vi "Process.vi"(8 "error in":errorcluster, 11 "Render.IMAQ":refnum<class "Render.IMAQ.lvclass">) -> (0 "error out":errorcluster, 3 "Render.IMAQ out":refnum<class "Render.IMAQ.lvclass">)   [LabVIEW 2019, in "Render.IMAQ.lvclass"]
doc: "---------------------------------------------------------------\nJKI State Machine Objects™\nhttp://jki.net/state-machine-objects/\nCopyright (C) 2005-2015, JKI <info@jki.net>\nALL RIGHTS RESERVED"
uses:
  Render.IMAQ.lvclass
  C:/Program Files (x86)/National Instruments/LabVIEW 2019/vi.lib/JKI/JKI SMO/SMO/SMO.lvclass
  <userlib>/LevyLab/Relay Box/Typedefs/Resistor--enum.ctl
  <vilib>/JKI/JKI SMO/SMO/Typedefs/Parent Call--Enum.ctl
  <vilib>/vision/Image Controls.llb/IMAQ Image.ctl
  <vilib>/JKI/JKI SMO/SMO/SMO.lvclass/SMO.ctl
  Render.IMAQ.lvclass/Render.IMAQ.ctl
  <vilib>/JKI/JKI SMO/SMO/Private/ReftoDVR--SMO.vi
  <vilib>/JKI/JKI SMO/SMO/SMO.lvclass
  <userlib>/LevyLab/Relay Box/Relay-Box.lvclass
panel:
  out "Array 2":T2(array[cluster])
  out "New Litho Data":T2(array[cluster])
  out "Array":bool[](array[boolean])
  # "For instructions on how to use the JKI State Machine Objects, examples and video tutorials, visit:\nhttp://jki.net/state-machine-objects/\n\nJKI State Machine Objects™\nhttp://jki.net/state-machine-objects/\nCopyright (C) 2005-2015, JKI <info@jki.net>\nALL RIGHTS RESERVED"
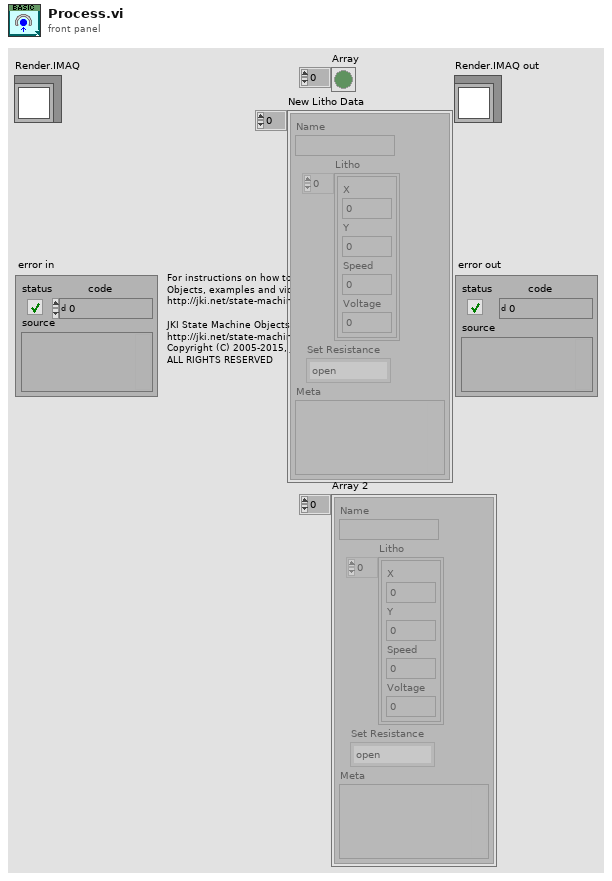
[diagram p1: front panel]
types:
  T1 = typedef "Relay-Box.lvclass/Resistor--enum.ctl" = enum16{"open", "discharge tip", "0 ohms", "100k ohm", "10M ohm", "1G ohm"}
  T2 = cluster{"Name":string, "Litho":cluster{"X":dbl, "Y":dbl, "Speed":dbl, "Voltage":dbl}[], "Set Resistance":T1, "Meta":variant}[]
  T3 = typedef "SMO.lvclass/Parent Call--Enum.ctl" = enum16{"Allows parent to run", "Does not request parent to run"}
  T4 = enum32{"invalid app kind", "Development System", "Run Time System", "Student Edition", "Embedded LabVIEW", "Evaluation", "Custom"}
  T5 = enum32{"Invalid", "Standard", "Closed", "Hidden", "Minimized", "Maximized"}
  T6 = enum32{"Bad", "Idle", "Run top level", "Running"}
  T7 = typedef "Render.IMAQ.lvclass/PrivateEvents--Render.IMAQ.New Background Image.ctl" = path
  T8 = typedef "IMAQ Image.ctl" = refnum<image>
  T9 = cluster{"Core":cluster{"Current VI Reference":refnum<vi>, "Close Panel on Exit?":bool, "error":errorcluster}, "Self Reference":refnum<class "Render.IMAQ.lvclass">, "Your string data":string, "Litho Data":cluster{"Name":string, "Litho":cluster{"X":dbl, "Y":dbl, "Speed":dbl, "Voltage":dbl}[], "Set Resistance":T1, "Meta":variant}[], "New Litho Data":cluster{"Name":string, "Litho":cluster{"X":dbl, "Y":dbl, "Speed":dbl, "Voltage":dbl}[], "Set Resistance":T1, "Meta":variant}[], "Background Path":path, "Changed":cluster{"Found":bool[], "Data":cluster{"Name":string, "Litho":cluster{"X":dbl, "Y":dbl, "Speed":dbl, "Voltage":dbl}[], "Set Resistance":T1, "Meta":variant}[]}, "IMAQ Work":T8}
  T10 = typedef "Render.IMAQ.lvclass/PrivateEvents--Render.IMAQ.NewLithographyData.ctl" = variant
  T11 = cluster{"Found":bool[], "Data":cluster{"Name":string, "Litho":cluster{"X":dbl, "Y":dbl, "Speed":dbl, "Voltage":dbl}[], "Set Resistance":T1, "Meta":variant}[]}
  T12 = cluster{"Current VI Reference":refnum<vi>, "Close Panel on Exit?":bool, "error":errorcluster}
  T13 = typedef "SMO.lvclass/Protected Events.ctl" = cluster{"StopProcesses":refnum<user-event>, "AbortProcesses":refnum<user-event>, "Config Changed":refnum<user-event>, "Dependency":refnum<user-event>}
  T14 = typedef "Render.IMAQ.lvclass/PrivateEvents--Cluster.ctl" = cluster{"New Background Image":refnum<user-event>, "NewLithographyData":refnum<user-event>}
  T15 = cluster{"Name":string, "Litho":cluster{"X":dbl, "Y":dbl, "Speed":dbl, "Voltage":dbl}[], "Set Resistance":T1, "Meta":variant}
  T16 = typedef "Image Type" = u32
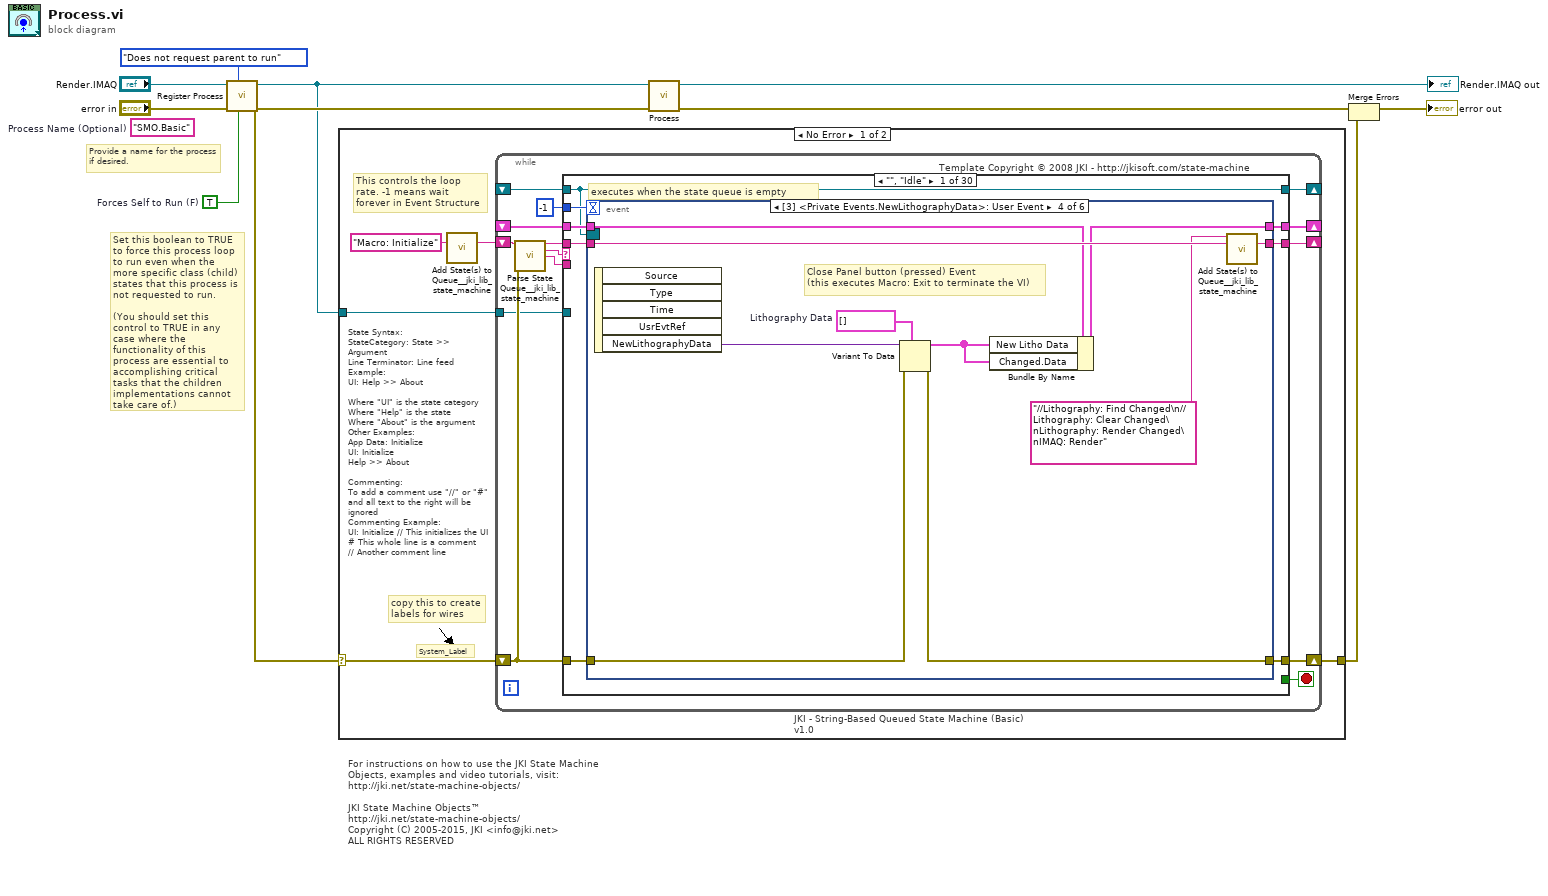
[diagram p0: block diagram]
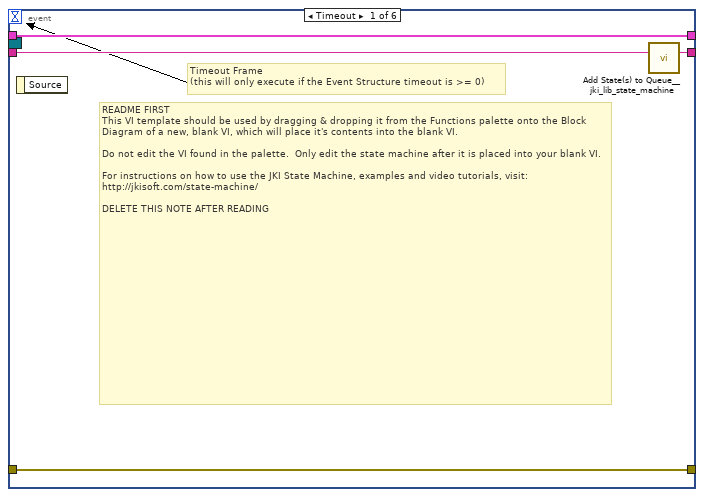
[diagram p2: hidden frame]
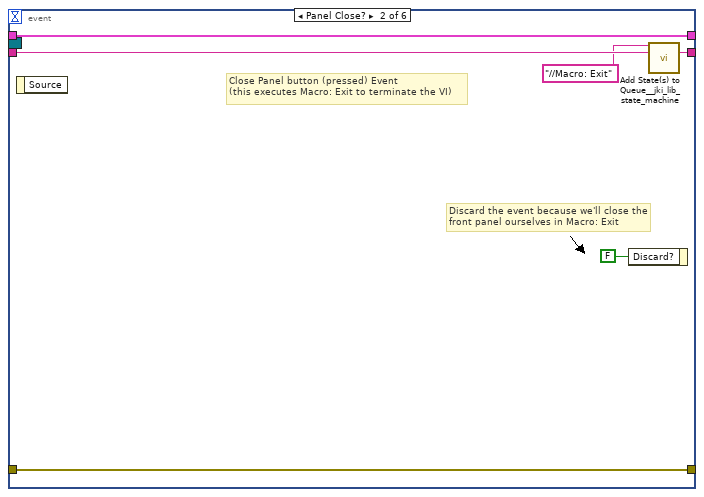
[diagram p3: hidden frame]
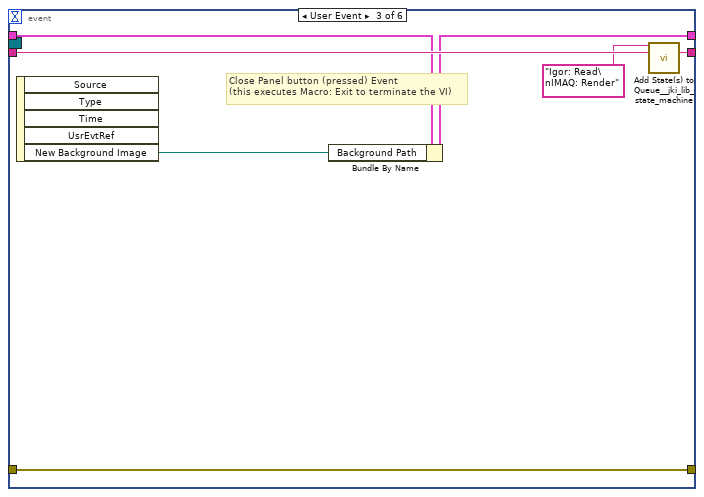
[diagram p4: hidden frame]
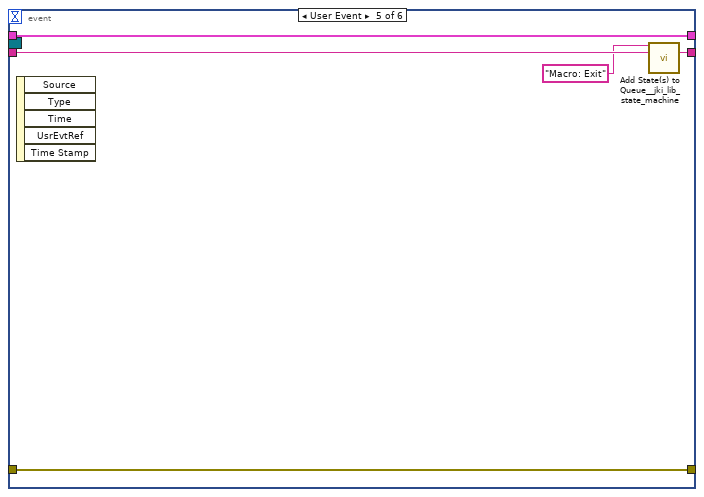
[diagram p5: hidden frame]
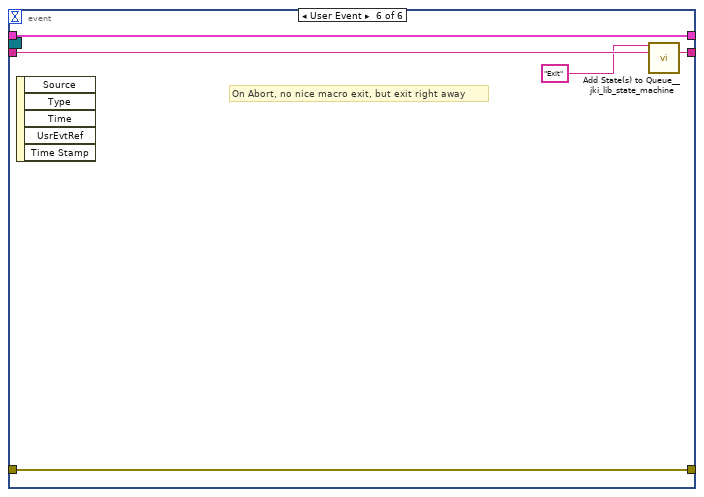
[diagram p6: hidden frame]
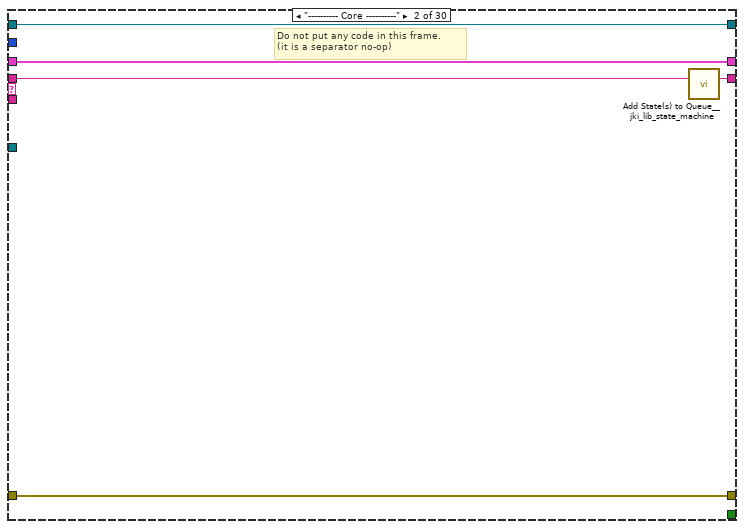
[diagram p7: hidden frame]
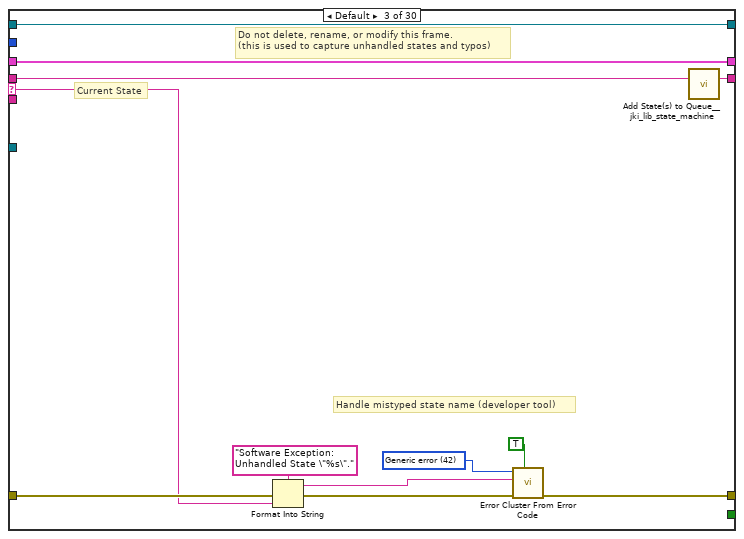
[diagram p8: hidden frame]
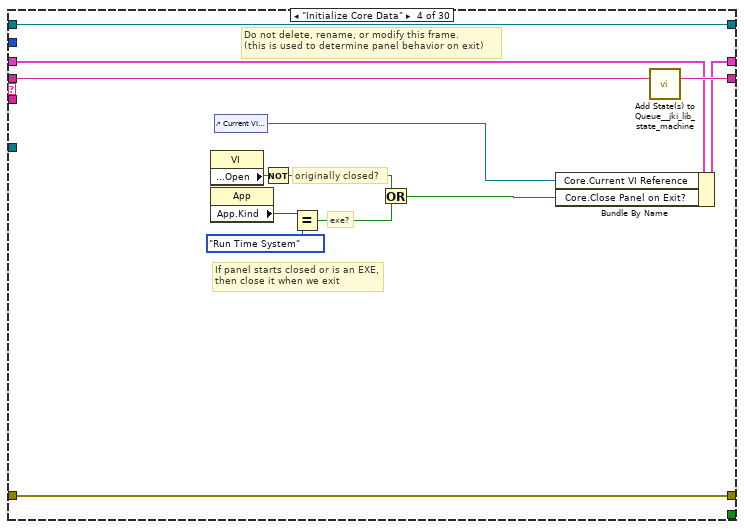
[diagram p9: hidden frame]
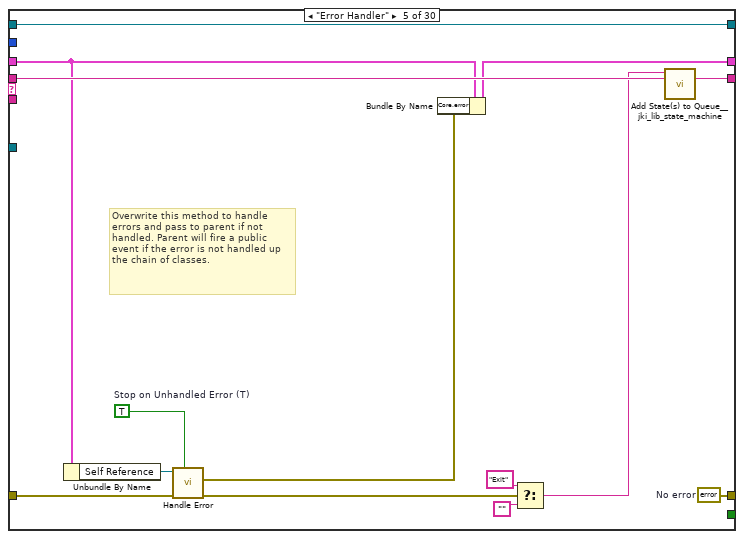
[diagram p10: hidden frame]
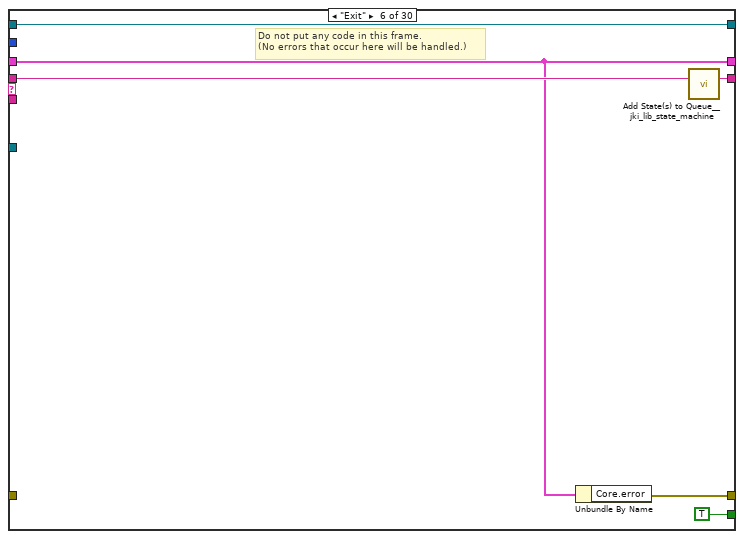
[diagram p11: hidden frame]
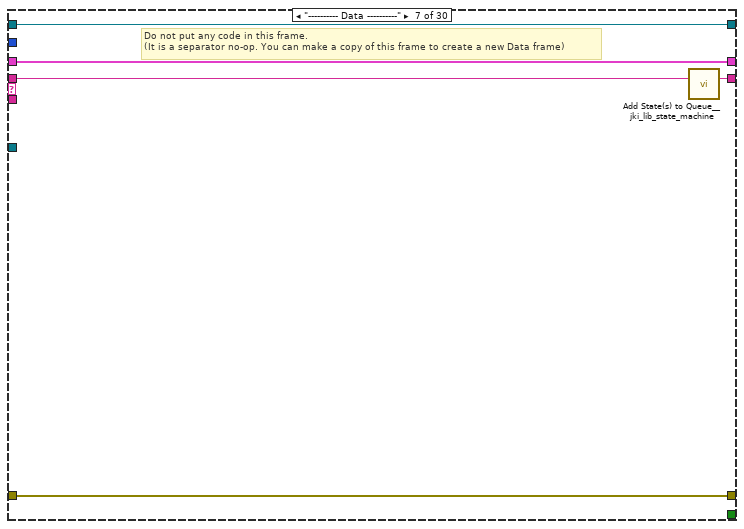
[diagram p12: hidden frame]
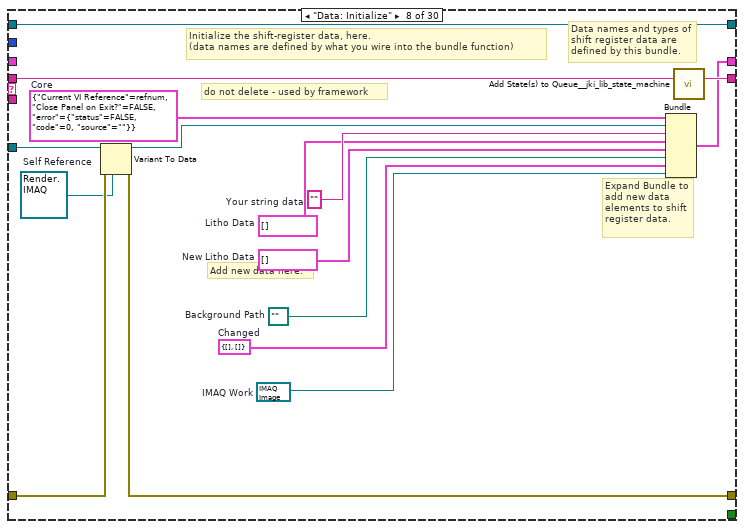
[diagram p13: hidden frame]
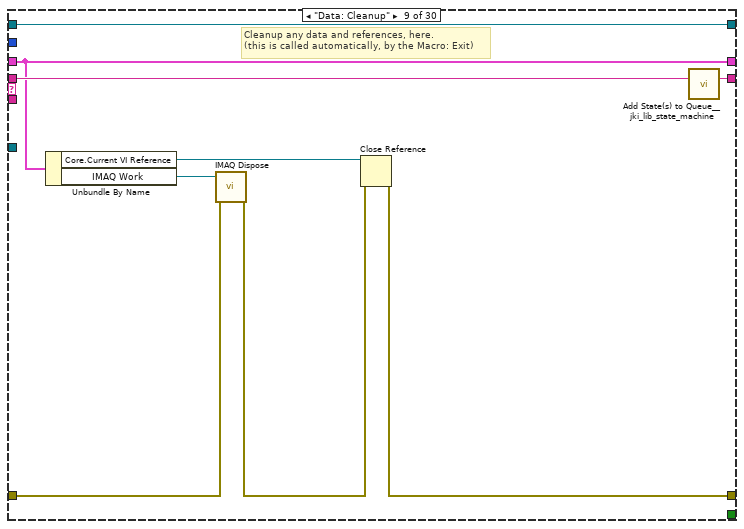
[diagram p14: hidden frame]
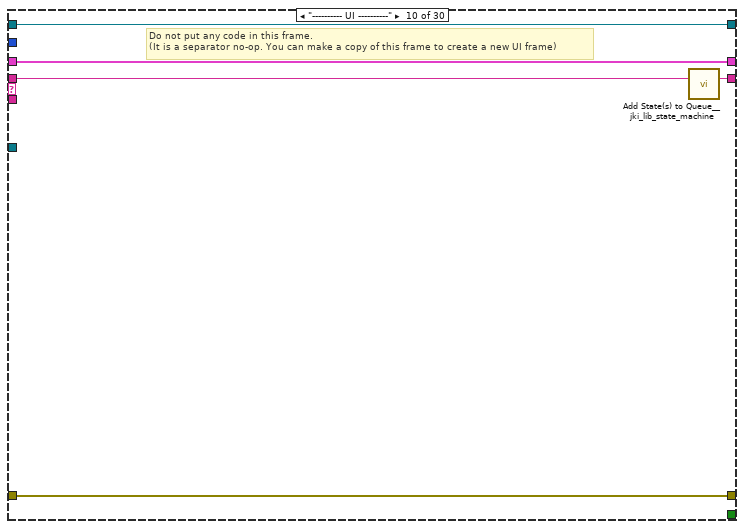
[diagram p15: hidden frame]
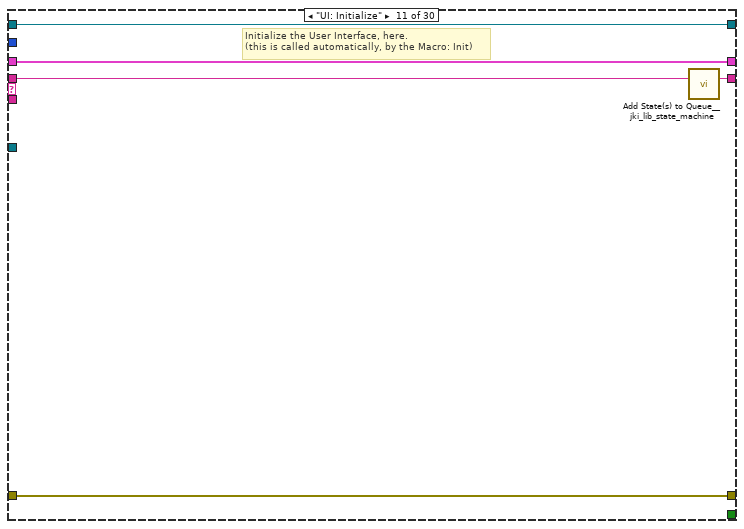
[diagram p16: hidden frame]
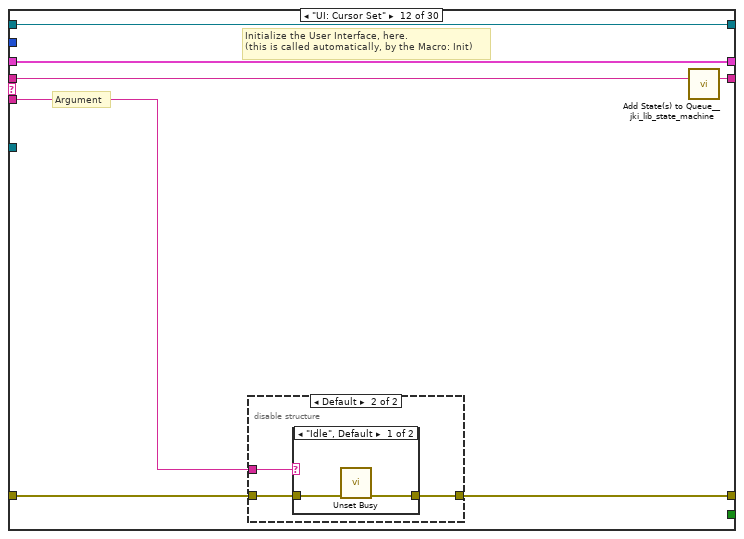
[diagram p17: hidden frame]
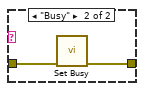
[diagram p19: hidden frame]
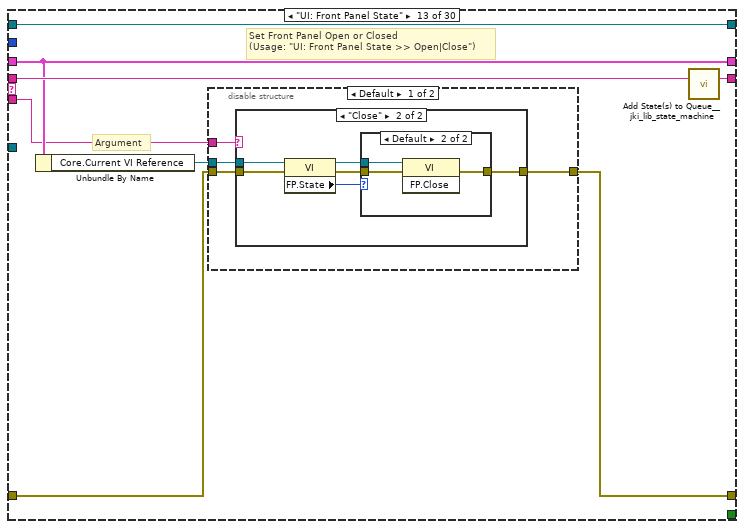
[diagram p20: hidden frame]
diagram:
  w1 = TRUE  # Forces Self to Run (F)
  (unwired) "SMO.Basic"  # Process Name (Optional)
  # "Provide a name for the process\nif desired."
  # "Set this boolean to TRUE to force this process loop to run even when the more specific class (child) states that this process is not requested to run.\n\n(You should set this control to TRUE in any case where the functionality of this process are essential to accomplishing critical tasks that the children implementations cannot take care of.)"
  # "For instructions on how to use the JKI State Machine Objects, examples and video tutorials, visit:\nhttp://jki.net/state-machine-objects/\n\nJKI State Machine Objects™\nhttp://jki.net/state-machine-objects/\nCopyright (C) 2005-2015, JKI <info@jki.net>\nALL RIGHTS RESERVED"
  n1 = call <vilib>:"Register Process.vi"("Forces Self to Run (F)"=w1, "Parent Call"=Parent_Call--Enum."Does not request parent to run", "error in (no error)"="error in", "SMO"="Render.IMAQ") -> ("error out"=w7:errorcluster, "SMO out"=w6:refnum<class "Render.IMAQ.lvclass">)  [unwired: 6 in]
  n2 = case shown="No Error" w7 {
    selector: w7 -> [w12 w397]
    tunnel: w6 -> [w13 _]
    tunnel: [w11 w397] -> w3
    frame No Error {
      # "State Syntax:\nStateCategory: State >> Argument\nLine Terminator: Line feed\nExample:\nUI: Help >> About\n\nWhere \"UI\" is the state category\nWhere \"Help\" is the state\nWhere \"About\" is the argument\nOther Examples:\nApp Data: Initialize\nUI: Initialize\nHelp >> About\n\nCommenting:\nTo add a comment use \"//\" or \"#\" and all text to the right will be ignored\nCommenting Example:\nUI: Initialize // This initializes the UI\n# This whole line is a comment\n// Another comment line"
      # "copy this to create labels for wires"
      # "This controls the loop rate. -1 means wait forever in Event Structure"
      # "System_Label"
      n3 = call <vilib>:"Add State(s) to Queue__jki_lib_state_machine.vi"("State(s) in (\"\")"="Macro: Initialize") -> ("States Out"=w15:string)  [unwired: 14 in]
      n4 = while "JKI - String-Based Queued State Machine (Basic) v1.0" {
        shift-right: [w22] -> _
        shift-left: _ -> [w21]
        shift-right: [w25] -> w11
        shift-left: w12 -> [w19]
        shift-right: [w24] -> _
        shift-left: w15 -> [w26]
        tunnel: w13 -> [w18]
        shift-right: [w17] -> _
        shift-left: _ -> [w16]
        stop <- w23 stop-if-true
        # "Template Copyright © 2008 JKI - http://jkisoft.com/state-machine"
        n5 = call <vilib>:"Parse State Queue__jki_lib_state_machine.vi"("State Queue"=w26, "Error In (no error)"=w19) -> ("Remaining States"=w28:string, "Current State"=w29:string, "Arguments"=w27:string)  [unwired: 11 in]
        n6 = case shown="\"\", \"Idle\"" w29 {
          selector: w29 -> [_ _ w81 _ _ _ _ _ _ _ _ _ _ _ _ _ _ _ _ _ _ _ _ _ _ _ _ _ _ _]
          tunnel: w28 -> [w37 w79 w85 w104 w118 w124 w129 w145 w154 w159 w164 w171 w187 w219 w233 w247 w252 w263 w268 w280 w286 w291 w303 w314 w344 w359 w369 w378 w383 w396]
          tunnel: w27 -> [_ _ _ _ _ _ _ _ _ _ _ w165 w181 _ _ _ _ _ _ _ _ _ _ _ _ _ _ _ _ _]
          tunnel: w21 -> [w35 w76 w83 w95 w112 w120 w126 _ w150 w156 w162 w169 w183 w216 w229 w238 w249 w260 w265 w278 w284 w289 w295 w309 w336 w357 w360 w375 w381 w386]
          tunnel: [w34 w77 w87 w101 w113 w119 w127 w140 w151 w157 w161 w166 w184 w217 w231 w245 w250 w254 w266 w274 w282 w287 w294 w311 w339 w355 w365 w370 w379 w392] -> w25
          tunnel: w19 -> [w33 w77 w86 w101 w114 _ w127 w141 w146 w157 w161 w167 w185 w217 w231 w245 w250 w255 w266 w275 w282 w287 w293 w311 w338 w355 w364 w371 w379 w391]
          tunnel: [w36 w78 w84 w103 w117 w123 w128 w144 w153 w158 w163 w170 w186 w218 w232 w246 w251 w262 w267 w279 w285 w290 w302 w313 w343 w358 w368 w377 w382 w395] -> w24
          tunnel: [_ _ _ _ _ TRUE _ _ _ _ _ _ _ _ _ _ _ _ _ _ _ _ _ _ _ _ _ _ _ _] -> w23
          tunnel: [w32 w76 w83 w102 w111 w120 w126 w143 w150 w156 w162 w169 w183 w216 w229 w238 w249 w260 w265 w278 w284 w289 w296 w310 w337 w357 w361 w375 w381 w387] -> w22
          tunnel: -1 ("Timeout") -> [w31 _ _ _ _ _ _ _ _ _ _ _ _ _ _ _ _ _ _ _ _ _ _ _ _ _ _ _ _ _]
          tunnel: w18 -> [_ _ _ _ _ _ _ w138 _ _ _ _ _ _ _ _ _ _ _ _ _ _ _ _ _ _ _ _ _ _]
          tunnel: [w30 w75 w80 w92 w116 w121 w125 w136 w149 w155 w160 w168 w180 w215 w230 w239 w248 w261 w264 w277 w283 w288 w301 w312 w342 w356 w367 w376 w380 w394] -> w17
          tunnel: w16 -> [w30 w75 w80 w92 w116 w121 w125 w136 w149 w155 w160 w168 w180 w215 w230 w239 w248 w261 w264 _ w283 w288 w301 w312 w342 w356 w367 w376 w380 w394]
          frame "", "Idle" {
            # "executes when the state queue is empty"
            n7 = event shown="[3] <Private Events.NewLithographyData>: User Event" {
              selector: w30 -> [_ _ _ _ _ _]
              dyn-events: _ -> [_ _ _ _ _ _]
              timeout: w31 -> [_ _ _ _ _ _]
              tunnel: w37 -> [w41 w47 w54 w64 w69 w74]
              tunnel: [w40 w46 w53 w63 w68 w73] -> w36
              tunnel: w35 -> [w39 w44 w49 w56 w66 w71]
              tunnel: [w38 w45 w52 w60 w67 w72] -> w34
              tunnel: w33 -> [w38 w45 w52 w59 w67 w72]
              tunnel: [w39 w44 w50 w57 w66 w71] -> w32
              event Timeout {
                # "README FIRST\nThis VI template should be used by dragging & dropping it from the Functions palette onto the Block Diagram of a new, blank VI, which will place it's contents into the blank VI.\n\nDo not edit the VI found in the palette.  Only edit the state machine after it is placed into your blank VI.\n\nFor instructions on how to use the JKI State Machine, examples and video tutorials, visit:\nhttp://jkisoft.com/state-machine/\n\nDELETE THIS NOTE AFTER READING"
                # "Timeout Frame\n(this will only execute if the Event Structure timeout is >= 0)"
                n8 = event-data() -> ()  [unwired: 1 in, 1 out]
                n9 = call <vilib>:"Add State(s) to Queue__jki_lib_state_machine.vi"("State(s) in (\"\")"=w41) -> ("States Out"=w40:string)  [unwired: 14 in]
              }
              event Panel Close? {
                # "Discard the event because we'll close the front panel ourselves in Macro: Exit"
                # "Close Panel button (pressed) Event\n(this executes Macro: Exit to terminate the VI)"
                n10 = event-data() -> ()  [unwired: 1 in, 1 out]
                n11 = event-data("Discard?"=FALSE) -> ()  [unwired: 1 in, 1 out]
                n12 = call <vilib>:"Add State(s) to Queue__jki_lib_state_machine.vi"("State(s) in Front (\"\")"="//Macro: Exit", "State(s) in (\"\")"=w47) -> ("States Out"=w46:string)  [unwired: 13 in]
              }
              event User Event {
                # "Close Panel button (pressed) Event\n(this executes Macro: Exit to terminate the VI)"
                n13 = event-data() -> ("New Background Image"=w48:T7)  [unwired: 1 in, 4 out]
                n14 = Bundle By Name(cluster=w49, "Background Path"=w48) -> (w50:T9)
                n15 = call <vilib>:"Add State(s) to Queue__jki_lib_state_machine.vi"("State(s) in Front (\"\")"="Igor: Read\nIMAQ: Render", "State(s) in (\"\")"=w54) -> ("States Out"=w53:string)  [unwired: 13 in]
              }
              event User Event {
                w58 = T2 []  # Lithography Data
                # "Close Panel button (pressed) Event\n(this executes Macro: Exit to terminate the VI)"
                n16 = event-data() -> ("NewLithographyData"=w61:T10)  [unwired: 1 in, 4 out]
                n17 = Variant To Data(error in=w59, type=w58, Variant=w61) -> (data=w55:T2, error out=w60:errorcluster)
                n18 = Bundle By Name(cluster=w56, "New Litho Data"=w55, "Changed.Data"=w55) -> (w57:T9)
                n19 = call <vilib>:"Add State(s) to Queue__jki_lib_state_machine.vi"("State(s) in Front (\"\")"="//Lithography: Find Changed\n//Lithography: Clear Changed\nLithography: Render Changed\nIMAQ: Render", "State(s) in (\"\")"=w64) -> ("States Out"=w63:string)  [unwired: 13 in]
              }
              event User Event {
                n20 = event-data() -> ()  [unwired: 1 in, 5 out]
                n21 = call <vilib>:"Add State(s) to Queue__jki_lib_state_machine.vi"("State(s) in Front (\"\")"="Macro: Exit", "State(s) in (\"\")"=w69) -> ("States Out"=w68:string)  [unwired: 13 in]
              }
              event User Event {
                # "On Abort, no nice macro exit, but exit right away"
                n22 = event-data() -> ()  [unwired: 1 in, 5 out]
                n23 = call <vilib>:"Add State(s) to Queue__jki_lib_state_machine.vi"("State(s) in Front (\"\")"="Exit", "State(s) in (\"\")"=w74) -> ("States Out"=w73:string)  [unwired: 13 in]
              }
            }
          }
          frame "---------- Core ----------" {
            # "Do not put any code in this frame.\n(it is a separator no-op)"
            n24 = call <vilib>:"Add State(s) to Queue__jki_lib_state_machine.vi"("State(s) in (\"\")"=w79) -> ("States Out"=w78:string)  [unwired: 14 in]
          }
          frame Default {
            w90 = 42 items=["No error", "Argument error", "Memory is full", "Out of zone", "End of file", "File already open", "Generic file I/O error", "File not found", "File permission error", "Disk is full", "Duplicate path", "Too many files open", "System feature not enabled", "Resource file not found", "Cannot add resource", "Resource not found", "Image not found", "Image memory error", "Pen does not exist", "Config type invalid", "Config token not found", "Config parse error", "Config memory error", "Bad external code format", "Bad external code offset", "External code not present", "Null window", "Destroy window error", "Null menu", "Print aborted", "Bad print record", "Print driver error", "Windows error during printing", "Memory error during printing", "Print dialog error", "Generic print error", "Invalid device refnum", "Device not found", "Device parameter error", "Device unit error", "Cannot open device", "Device call aborted", "Generic error", "Cancelled by user", "Object ID too low", "Object ID too high", "Object not in heap", "Unknown heap", "Unknown object (invalid DefProc)", "Unknown object (DefProc not in table)", "Message out of range", "Invalid (null) method", "Unknown message", "Manager call not supported", "Bad address", "Network operation in progress", "Network operation timed out", "Connection is busy", "Network attribute not supported", "Network error", "Address in use", "System out of memory", "Connection aborted", "Connection refused", "Not connected", "Already connected", "Connection closed", "Initialization error (interapplication manager)", "Bad occurrence", "Wait on unbound occurrence handler", "Occurrence queue overflow", "Datalog type conflict", "Unused", "Unrecognized type (interapplication manager)", "Memory corrupt", "Failed to make temporary DLL", "Old CIN version", "Drag socket not found", "Failed to load drop-object", "Failed to register OLE object", "Failed to release OLE object", "Format specifier type mismatch", "Unknown format specifier", "Too few format specifiers", "Too many format specifiers", "Scan failed", "Newer CIN version", "Error converting to variant", "Runtime menu error", "Password tampered", "Variant attribute not found", "Incompatible variant data type", "Event data is not available", "Event Store is not present", "Occurrence is not found", "Event Queue is not created", "Event info is not available", "Refnum passed is NULL", "Error retrieving Class GUID", "Error retrieving CoClass GUID", "Error retrieving TypeLib GUID.", "Bad built application magic bytes.", "Specific driver is different from the specific driver associated with the Logical Name.", "There is no session opened to the class driver.", "Max Error", "MAX - Error with config objects", "MAX - Error loading configuration", "MAX - Group not supported"]
            # "Current State"
            # "Do not delete, rename, or modify this frame.\n(this is used to capture unhandled states and typos)"
            # "Handle mistyped state name (developer tool)"
            n25 = Format Into String(format string="Software Exception: Unhandled State \"%s\"." ("message"), error in=w86, w81) -> (resulting string=w89:string, error out=w88:errorcluster)  [unwired: 1 in]
            n26 = call <vilib>:"Error Cluster From Error Code.vi"("show call chain? (False)"=TRUE, "error in (no error)"=w88, "error message (\"\")"=w89, "error code (0)"=w90) -> ("error out"=w87:errorcluster)  [unwired: 5 in]
            n27 = call <vilib>:"Add State(s) to Queue__jki_lib_state_machine.vi"("State(s) in (\"\")"=w85) -> ("States Out"=w84:string)  [unwired: 14 in]
          }
          frame "Initialize Core Data" {
            # "Do not delete, rename, or modify this frame.\n(this is used to determine panel behavior on exit)"
            # "originally closed?"
            # "exe?"
            # "If panel starts closed or is an EXE, then close it when we exit"
            n28 = property class="VI"() -> ("Front Panel.Open"=w100:bool)  [unwired: 2 in, 2 out]
            n29 = property class="App"() -> ("App.Kind"=w99:T4)  [unwired: 2 in, 2 out]
            n30 = control-ref of="Current VI Reference"() -> (w93:refnum<vi>)
            n31 = Not(x=w100) -> (.not. x?=w97:bool)
            n32 = Equal?(x=w99, y=T4."Run Time System" ("Application:Kind")) -> (x = y?=w96:bool)
            n33 = Or(x=w97, y=w96) -> (x .or. y?=w94:bool)
            n34 = Bundle By Name(cluster=w95, "Core.Current VI Reference"=w93, "Core.Close Panel on Exit?"=w94) -> (w102:T9)
            n35 = call <vilib>:"Add State(s) to Queue__jki_lib_state_machine.vi"("State(s) in (\"\")"=w104) -> ("States Out"=w103:string)  [unwired: 14 in]
          }
          frame "Error Handler" {
            w105 = TRUE  # Stop on Unhandled Error (T)
            w113 = errorcluster {"status"=FALSE, "code"=0, "source"=""}  # No error
            # "Overwrite this method to handle errors and pass to parent if not handled. Parent will fire a public event if the error is not handled up the chain of classes."
            n36 = Unbundle By Name(w112) -> ("Self Reference"=w115:refnum<class "Render.IMAQ.lvclass">)
            n37 = call-dynamic "Handle Error.vi"("Stop on Unhandled Error (T)"=w105, "error in"=w114, "SMO"=w115) -> ("handling error"=w106:errorcluster, "Unhandled error"=w109:errorcluster)  [unwired: 6 in, 1 out]
            n38 = Bundle By Name(cluster=w112, "Core.error"=w109) -> (w111:T9)
            n39 = Select(t="Exit", s=w106, f="") -> (s? t:f=w110:string)
            n40 = call <vilib>:"Add State(s) to Queue__jki_lib_state_machine.vi"("State(s) in Front (\"\")"=w110, "State(s) in (\"\")"=w118) -> ("States Out"=w117:string)  [unwired: 13 in]
          }
          frame "Exit" {
            # "Do not put any code in this frame.\n(No errors that occur here will be handled.)"
            n41 = Unbundle By Name(w120) -> ("Core.error"=w119:errorcluster)
            n42 = call <vilib>:"Add State(s) to Queue__jki_lib_state_machine.vi"("State(s) in (\"\")"=w124) -> ("States Out"=w123:string)  [unwired: 14 in]
          }
          frame "---------- Data ----------" {
            # "Do not put any code in this frame.\n(It is a separator no-op. You can make a copy of this frame to create a new Data frame)"
            n43 = call <vilib>:"Add State(s) to Queue__jki_lib_state_machine.vi"("State(s) in (\"\")"=w129) -> ("States Out"=w128:string)  [unwired: 14 in]
          }
          frame "Data: Initialize" {
            w130 = T11 {"Found"=[], "Data"=[]}  # Changed
            w131 = T8 refnum  # IMAQ Work
            w132 = path ""  # Background Path
            w133 = T2 []  # New Litho Data
            w134 = T2 []  # Litho Data
            w135 = T12 {"Current VI Reference"=refnum, "Close Panel on Exit?"=FALSE, "error"={"status"=FALSE, "code"=0, "source"=""}}  # Core
            w139 = refnum<class "Render.IMAQ.lvclass"> refnum  # Self Reference
            w142 = ""  # Your string data
            # "do not delete - used by framework"
            # "Expand Bundle to add new data elements to shift register data."
            # "Add new data here."
            # "Data names and types of shift register data are defined by this bundle."
            # "Initialize the shift-register data, here.\n(data names are defined by what you wire into the bundle function)"
            n44 = Variant To Data(error in=w141, type=w139, Variant=w138) -> (data=w137:refnum<class "Render.IMAQ.lvclass">, error out=w140:errorcluster)
            n45 = Bundle("Core"=w135, "Self Reference"=w137, "Your string data"=w142, "Litho Data"=w134, "New Litho Data"=w133, "Background Path"=w132, "Changed"=w130, "IMAQ Work"=w131) -> (w143:T9)  [unwired: 1 in]
            n46 = call <vilib>:"Add State(s) to Queue__jki_lib_state_machine.vi"("State(s) in (\"\")"=w145) -> ("States Out"=w144:string)  [unwired: 14 in]
          }
          frame "Data: Cleanup" {
            # "Cleanup any data and references, here.\n(this is called automatically, by the Macro: Exit)"
            n47 = Unbundle By Name(w150) -> ("Core.Current VI Reference"=w152:refnum<vi>, "IMAQ Work"=w148:T8)
            n48 = call "IMAQ Dispose"("Image"=w148, "error in (no error)"=w146) -> ("error out"=w147:errorcluster)  [unwired: 4 in]
            n49 = Close Reference(reference=w152, error in (no error)=w147) -> (error out=w151:errorcluster)
            n50 = call <vilib>:"Add State(s) to Queue__jki_lib_state_machine.vi"("State(s) in (\"\")"=w154) -> ("States Out"=w153:string)  [unwired: 14 in]
          }
          frame "---------- UI ----------" {
            # "Do not put any code in this frame.\n(It is a separator no-op. You can make a copy of this frame to create a new UI frame)"
            n51 = call <vilib>:"Add State(s) to Queue__jki_lib_state_machine.vi"("State(s) in (\"\")"=w159) -> ("States Out"=w158:string)  [unwired: 14 in]
          }
          frame "UI: Initialize" {
            # "Initialize the User Interface, here.\n(this is called automatically, by the Macro: Init)"
            n52 = call <vilib>:"Add State(s) to Queue__jki_lib_state_machine.vi"("State(s) in (\"\")"=w164) -> ("States Out"=w163:string)  [unwired: 14 in]
          }
          frame "UI: Cursor Set" {
            # "Argument"
            # "Initialize the User Interface, here.\n(this is called automatically, by the Macro: Init)"
            n53 = disable-structure shown="Default" {
              disable-tunnel: w167 -> [w172 w175]
              disable-tunnel: [w172 w174] -> w166
              disable-tunnel: w165 -> [_ w173]
              frame condition #0 {
              }
              frame condition #1 (active) {
                n54 = case shown="\"Idle\", Default" w173 {
                  tunnel: w175 -> [w177 w179]
                  tunnel: [w176 w178] -> w174
                  frame "Idle", Default {
                    n55 = call <vilib>:"Unset Busy.vi"("error in (no error)"=w177) -> ("error out"=w176:errorcluster)  [unwired: 10 in]
                  }
                  frame "Busy" {
                    n56 = call <vilib>:"Set Busy.vi"("error in (no error)"=w179) -> ("error out"=w178:errorcluster)  [unwired: 9 in, 1 out]
                  }
                }
              }
            }
            n57 = call <vilib>:"Add State(s) to Queue__jki_lib_state_machine.vi"("State(s) in (\"\")"=w171) -> ("States Out"=w170:string)  [unwired: 14 in]
          }
          frame "UI: Front Panel State" {
            # "Argument"
            # "Set Front Panel Open or Closed\n(Usage: \"UI: Front Panel State >> Open|Close\")"
            n58 = Unbundle By Name(w183) -> ("Core.Current VI Reference"=w182:refnum<vi>)
            n59 = disable-structure shown="Default" {
              disable-tunnel: w185 -> [w191 w214]
              disable-tunnel: [w190 w214] -> w184
              disable-tunnel: w182 -> [w189 _]
              disable-tunnel: w181 -> [w188 _]
              frame condition #0 (active) {
                n60 = case shown="\"Close\"" w188 {
                  tunnel: w191 -> [w195 w208]
                  tunnel: [w197 w209] -> w190
                  tunnel: w189 -> [w196 w206]
                  frame "Open", Default {
                    n61 = property class="VI"(reference=w196, error in=w195) -> (reference out=w193:refnum<vi>, error out=w194:errorcluster, "FP.State"=w192:T5)
                    n62 = case shown="\"Closed\"" w192 {
                      tunnel: [w200 w203] -> w197
                      tunnel: w194 -> [w199 w203]
                      tunnel: w193 -> [w198 _]
                      frame "Closed" {
                        n63 = invoke class="VI" method="FP.Open"(reference=w198, error in=w199, "Activate"=TRUE, "State"=T5."Standard") -> (error out=w200:errorcluster)  [unwired: 1 in, 4 out]
                      }
                      frame Default {
                      }
                    }
                  }
                  frame "Close" {
                    n64 = property class="VI"(reference=w206, error in=w208) -> (reference out=w205:refnum<vi>, error out=w207:errorcluster, "FP.State"=w204:T5)
                    n65 = case shown="Default" w204 {
                      tunnel: [w210 w213] -> w209
                      tunnel: w207 -> [w210 w212]
                      tunnel: w205 -> [_ w211]
                      frame "Invalid", "Closed" {
                      }
                      frame Default {
                        n66 = invoke class="VI" method="FP.Close"(reference=w211, error in=w212) -> (error out=w213:errorcluster)  [unwired: 1 in, 2 out]
                      }
                    }
                  }
                }
              }
              frame condition #1 {
              }
            }
            n67 = call <vilib>:"Add State(s) to Queue__jki_lib_state_machine.vi"("State(s) in (\"\")"=w187) -> ("States Out"=w186:string)  [unwired: 14 in]
          }
          frame "---------- Macro ----------" {
            # "Do not put any code in this frame.\n(It is a separator no-op. You can make a copy of this frame to create a new Macro frame)"
            n68 = call <vilib>:"Add State(s) to Queue__jki_lib_state_machine.vi"("State(s) in (\"\")"=w219) -> ("States Out"=w218:string)  [unwired: 14 in]
          }
          frame "Macro: Initialize" {
            w224 = "UI: Initialize\nUI: Front Panel State >> Open\nIMAQ: Init"  # UI: Initialize UI: Front Panel State >> Open IMAQ: Init
            w220 = "Process: Sync"
            # "Initialization Macro\n(This is called once, when the VI starts)"
            n69 = control-ref of="This VI"() -> (w222:refnum<vi>)
            n70 = property class="VI"(reference=w222) -> ("Exec.State"=w221:T6)  [unwired: 1 in, 2 out]
            n71 = Equal?(x=w221, y=T6."Run top level") -> (x = y?=w227:bool)
            n72 = Select(t=w220, s=w227, f="") -> ()  [unwired: 1 out]
            n73 = call <vilib>:"Add State(s) to Queue__jki_lib_state_machine.vi"("State(s) in Front (\"\")"="Data: Initialize\nInitialize Core Data\nEvents: Register", "State(s) in (\"\")"=w220, "State(s) at Back (\"\")"=w224) -> ("States Out"=w223:string)  [unwired: 12 in]
            n74 = call <vilib>:"Add State(s) to Queue__jki_lib_state_machine.vi"("State(s) in Front (\"\")"=w223, "State(s) in (\"\")"=w233) -> ("States Out"=w232:string)  [unwired: 13 in]
          }
          frame "Macro: Exit" {
            # "Exit Macro\n(This is called once, when the VI exits)"
            n75 = Unbundle By Name(w238) -> ("Core.Close Panel on Exit?"=w244:bool)
            n76 = Select(t="UI: Front Panel State >> Close", s=w244, f="") -> (s? t:f=w241:string)
            n77 = call <vilib>:"Add State(s) to Queue__jki_lib_state_machine.vi"("State(s) in Front (\"\")"="Data: Cleanup\nEvents: Unregister", "State(s) in (\"\")"="Process: Sync", "State(s) at Back (\"\")"="Exit") -> ("States Out"=w235:string)  [unwired: 12 in]
            n78 = call <vilib>:"Add State(s) to Queue__jki_lib_state_machine.vi"("State(s) in (\"\")"=w241, "State(s) at Back (\"\")"=w235) -> ("States Out"=w240:string)  [unwired: 13 in]
            n79 = call <vilib>:"Add State(s) to Queue__jki_lib_state_machine.vi"("State(s) in Front (\"\")"=w240, "State(s) in (\"\")"=w247) -> ("States Out"=w246:string)  [unwired: 13 in]
          }
          frame "---------- Process ----------" {
            # "Template Separator\n(You can make a copy of, or modify, this frame)"
            n80 = call <vilib>:"Add State(s) to Queue__jki_lib_state_machine.vi"("State(s) in (\"\")"=w252) -> ("States Out"=w251:string)  [unwired: 14 in]
          }
          frame "Process: Sync" {
            n81 = Unbundle By Name(w260) -> ("Self Reference"=w256:refnum<class "Render.IMAQ.lvclass">)
            n82 = call <vilib>:"WaitOnProcessSync.vi"("error in (no error)"=w255, "SMO"=w256) -> ("error out"=w254:errorcluster, "Don't run?"=w259:bool)  [unwired: 7 in, 1 out]
            n83 = Select(t="Data: Cleanup\nEvents: Unregister\nExit", s=w259, f="") -> (s? t:f=w253:string)
            n84 = call <vilib>:"Add State(s) to Queue__jki_lib_state_machine.vi"("State(s) in Front (\"\")"=w253, "State(s) in (\"\")"=w263) -> ("States Out"=w262:string)  [unwired: 13 in]
          }
          frame "---------- Events ----------" {
            # "Template Separator\n(You can make a copy of, or modify, this frame)"
            n85 = call <vilib>:"Add State(s) to Queue__jki_lib_state_machine.vi"("State(s) in (\"\")"=w268) -> ("States Out"=w267:string)  [unwired: 14 in]
          }
          frame "Events: Register" {
            # "Expand to add\nmore events"
            n86 = Unbundle By Name(w278) -> ("Self Reference"=w271:refnum<class "Render.IMAQ.lvclass">)
            n87 = call <vilib>:"GetProtectedEvents.vi"("SMO"=w271) -> ("error out"=w272:errorcluster, "SMO Protected Events"=w276:T13)  [unwired: 8 in, 1 out]
            n88 = call "Render.IMAQ.GetPrivateEvents.vi"("Render.IMAQ"=w271) -> ("error out"=w269:errorcluster, "Private Events"=w270:T14)  [unwired: 8 in, 1 out]
            n89 = register-events(w276, w270) -> (reference out=w277:refnum<event-registration>, error out=w273:errorcluster)  [unwired: 2 in]
            n90 = Merge Errors(w275, w273, w272, w269) -> (w274:errorcluster)
            n91 = call <vilib>:"Add State(s) to Queue__jki_lib_state_machine.vi"("State(s) in (\"\")"=w280) -> ("States Out"=w279:string)  [unwired: 14 in]
          }
          frame "Events: Unregister" {
            n92 = Unregister For Events(event registration refnum=w283, error in=w282) -> (error out=w281:errorcluster)
            n93 = call <vilib>:"Clear Errors.vi"("error in (no error)"=w281) -> ()  [unwired: 5 in, 2 out]
            n94 = call <vilib>:"Add State(s) to Queue__jki_lib_state_machine.vi"("State(s) in (\"\")"=w286) -> ("States Out"=w285:string)  [unwired: 14 in]
          }
          frame "---------- Lithography ----------" {
            n95 = call <vilib>:"Add State(s) to Queue__jki_lib_state_machine.vi"("State(s) in (\"\")"=w291) -> ("States Out"=w290:string)  [unwired: 14 in]
          }
          frame "Lithography: Render Changed" {
            n96 = Unbundle By Name(w295) -> ("Changed.Data"=w298:T2, "IMAQ Work"=w299:T8)
            n97 = call "Image Generator.vi"("Hide Labels"=FALSE, "Lithography Data"=w298, "error in (no error)"=w293, "Resolution"=256, "Image Reference In"=w299) -> ("error out"=w294:errorcluster, "Image Reference Out"=w297:T8)  [unwired: 5 in]
            n98 = Bundle By Name(cluster=w295, "IMAQ Work"=w297) -> (w296:T9)
            n99 = call <vilib>:"Add State(s) to Queue__jki_lib_state_machine.vi"("State(s) in (\"\")"=w303) -> ("States Out"=w302:string)  [unwired: 14 in]
          }
          frame "Lithography: Find Changed" {
            n100 = Unbundle By Name(w309) -> ("Litho Data"=w307:T2, "New Litho Data"=w304:T2)
            "New Litho Data" <- w304
            n101 = for {
              tunnel: w307 -> [w331] mode=indexing
              tunnel: [w330] -> w308 mode=indexing
              n102 = Unbundle By Name(w331) -> ("Name"=w330:string)
            }
            n103 = for {
              tunnel: w308 -> [w322]
              tunnel: w304 -> [w319] mode=indexing
              tunnel: w307 -> [w320]
              tunnel: [w316] -> w306 mode=indexing if=w318
              tunnel: [w315] -> w305 mode=indexing
              n104 = Unbundle By Name(w319) -> ("Name"=w321:string)
              n105 = Search 1D Array(1D array=w322, element=w321) -> (index of element=w317:i32)  [unwired: 1 in]
              n106 = Greater Or Equal To 0?(x=w317) -> (x >= 0?=w315:bool)
              n107 = case shown="True" w315 {
                tunnel: w320 -> [_ w329]
                tunnel: w319 -> [w324 w325]
                tunnel: [TRUE w327] -> w318
                tunnel: w317 -> [_ w326]
                tunnel: [w324 w325] -> w316
                frame False {
                }
                frame True {
                  n108 = Index Array(array=w329, index=w326) -> (element=w328:T15)
                  n109 = Not Equal?(x=w328, y=w325) -> (x != y?=w327:bool)
                }
              }
            }
            "Array" <- w305
            "Array 2" <- w306
            n110 = Bundle By Name(cluster=w309, "Changed.Data"=w306, "Changed.Found"=w305, "Litho Data"=w304) -> (w310:T9)
            n111 = call <vilib>:"Add State(s) to Queue__jki_lib_state_machine.vi"("State(s) in (\"\")"=w314) -> ("States Out"=w313:string)  [unwired: 14 in]
          }
          frame "Lithography: Clear Changed" {
            n112 = Unbundle By Name(w336) -> ("Changed.Found"=w333:bool[], "Changed.Data"=w341:T2, "IMAQ Work"=w334:T8)
            n113 = Or Array Elements(Boolean array=w333) -> (logical OR=w332:bool)
            n114 = for {
              tunnel: w341 -> [w354] mode=indexing
              tunnel: [w353] -> w340 mode=indexing if=w352
              tunnel: w333 -> [w352] mode=indexing
              n115 = Unbundle By Name(w354) -> ("Name"=w353:string)
            }
            n116 = case shown="True" w332 {
              tunnel: w340 -> [_ w351]
              tunnel: [w345 w350] -> w339
              tunnel: w338 -> [w345 w349]
              tunnel: [w346 w348] -> w335
              tunnel: w334 -> [w346 w347]
              frame False {
              }
              frame True {
                n117 = call "IMAQ Clear Overlay"("Groups"=w351, "error in (no error)"=w349, "Image"=w347) -> ("error out"=w350:errorcluster, "Image Out"=w348:T8)  [unwired: 7 in]
              }
            }
            n118 = Bundle By Name(cluster=w336, "IMAQ Work"=w335) -> (w337:T9)
            n119 = call <vilib>:"Add State(s) to Queue__jki_lib_state_machine.vi"("State(s) in (\"\")"=w344) -> ("States Out"=w343:string)  [unwired: 14 in]
          }
          frame "---------- IMAQ ----------" {
            n120 = call <vilib>:"Add State(s) to Queue__jki_lib_state_machine.vi"("State(s) in (\"\")"=w359) -> ("States Out"=w358:string)  [unwired: 14 in]
          }
          frame "IMAQ: Init" {
            w366 = T16 2 items=["Grayscale (U8)", "Grayscale (I16)", "Grayscale (SGL)", "Complex (CSG)", "RGB (U32)", "HSL (U32)", "RGB (U64)", "Grayscale (U16)"] ("Image Type")
            n121 = call "Imaq Create"("Image Name"="Working", "Image Type"=w366, "error in (no error)"=w364) -> ("New Image"=w362:T8, "error out"=w365:errorcluster)  [unwired: 1 in, 1 out]
            n122 = Bundle By Name(cluster=w360, "IMAQ Work"=w362) -> (w361:T9)
            n123 = call <vilib>:"Add State(s) to Queue__jki_lib_state_machine.vi"("State(s) in (\"\")"=w369) -> ("States Out"=w368:string)  [unwired: 14 in]
          }
          frame "IMAQ: Render" {
            (unwired) 100 ("Y Resolution")
            n124 = Unbundle By Name(w375) -> ("IMAQ Work"=w374:T8, "Self Reference"=w372:refnum<class "Render.IMAQ.lvclass">)
            n125 = Unbundle By Name(w372) -> ("IMAQ.Ref"=w373:T8)
            n126 = call "IMAQ Copy"("error in (no error)"=w371, "Image Dst"=w373, "Image Src"=w374) -> ("error out"=w370:errorcluster)  [unwired: 3 in, 1 out]
            n127 = call <vilib>:"Add State(s) to Queue__jki_lib_state_machine.vi"("State(s) in (\"\")"=w378) -> ("States Out"=w377:string)  [unwired: 14 in]
          }
          frame "---------- Igor ----------" {
            n128 = call <vilib>:"Add State(s) to Queue__jki_lib_state_machine.vi"("State(s) in (\"\")"=w383) -> ("States Out"=w382:string)  [unwired: 14 in]
          }
          frame "Igor: Read" {
            n129 = Unbundle By Name(w386) -> ("Background Path"=w393:path)
            n130 = call "Background.vi"("Image data max"=100.0, "Image data min"=0.0, "error in (no error)"=w391, "Resolution"=256, "Page"=0, "Image File Path"=w393) -> ("error out"=w392:errorcluster, "Background out"=w388:T8)  [unwired: 2 in, 2 out]
            n131 = Bundle By Name(cluster=w386, "IMAQ Work"=w388) -> (w387:T9)
            n132 = call <vilib>:"Add State(s) to Queue__jki_lib_state_machine.vi"("State(s) in (\"\")"=w396) -> ("States Out"=w395:string)  [unwired: 14 in]
          }
        }
      }
    }
    frame Error {
    }
  }
  n133 = call-parent "Process.vi"("error in"=w7, "SMO"=w6) -> ("error out"=w4:errorcluster, "SMO out"=→"Render.IMAQ out":refnum<class "Render.IMAQ.lvclass">)  [unwired: 8 in]
  n134 = Merge Errors(w4, w3) -> (→"error out":errorcluster)
